vi "XYZ Stage Driver.vi"(11 "UI elements cluster":T1) -> (0 "error out (no error)":errorcluster)   [LabVIEW 2020]
uses:
  Global Variables/General Globals.vi
  Typedefs/HW config states enum.ctl
  Typedefs/XYZ stage states.ctl
  Global Variables/gl_UI Ctrl Refs.vi
  Globals/gl_XYZStage globals.vi
  Typedefs/Plane Mode.ctl
  Typedefs/Laser control knob.ctl
  Typedefs/PMT control knob.ctl
  Typedefs/XY Stage_Move.ctl
  Typedefs/Frame Size.ctl
  Typedefs/UI ctrl refs cluster.ctl
  Acquisition/Typedefs/Ref DAQ Param.ctl
  Typedefs/test_fpga_control.ctl
  User Interface/Misc/Biology Information.ctl
  User Interface/Misc/Experiment Type.ctl
panel:
  out "Interrupt loop itr":i32
  out "XYZ stage initialised":bool
  out "Motor driver loop itr":i32
  out "Command":T2
  out "Coordinates":cluster{"X":sgl, "Y":sgl, "Z":sgl}
  out "internal error cluster":errorcluster
  # "XYZ STAGE DRIVER"
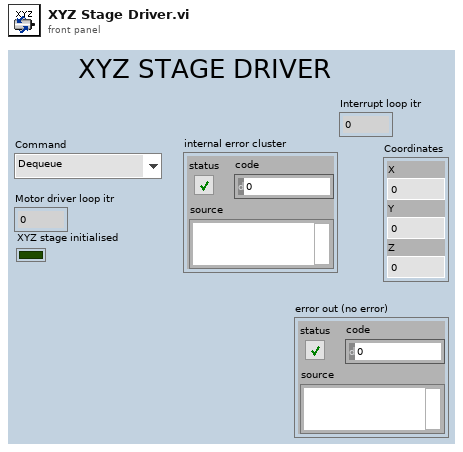
[diagram p1: front panel]
types:
  T1 = typedef "UI ctrl refs cluster.ctl" = cluster{"Top level VI path":path, "Top level VI ref":refnum<vi>, "User menu ref":refnum<k9>, "Sub Panel control":refnum<vi>, "Imaging Param Tab":refnum<vi>, "Occurrence-Start drivers":refnum<k4>, "Occurrence-Speed logging initialised":refnum<k4>, "Occurrence-XYZ stage initialised":refnum<k4>, "Exit button":refnum<vi>, "Status ind":refnum<vi>, "Set as origin":refnum<vi>, "Speed Logging":refnum<vi>, "Time Lapse":refnum<vi>, "Live Imaging":refnum<vi>, "AOL Z Stack":refnum<vi>, "Motor Z Stack":refnum<vi>, "Funct Acq button":refnum<vi>, "Hard Shutter":refnum<vi>, "Virtual Shutter":refnum<vi>, "Laser Power":refnum<vi>, "AOL Mode":refnum<vi>, "Frame Size":refnum<vi>, "Field of View":refnum<vi>, "Dwell Time":refnum<vi>, "Zoom":refnum<vi>, "AOL Z":refnum<vi>, "Objective":refnum<vi>, "Axis":refnum<vi>, "Paths & Names":refnum<vi>, "Experiment folder path (ind.)":refnum<vi>, "Last State (Ind.)":refnum<vi>, "Averages":refnum<vi>, "Angle (degrees)":refnum<vi>, "X centre":refnum<vi>, "Y centre":refnum<vi>, "Plane Mode":refnum<vi>, "# Planes":refnum<vi>, "Z Start":refnum<vi>, "Z Stop":refnum<vi>, "Z Step":refnum<vi>, "PMT 1":refnum<vi>, "PMT 2":refnum<vi>, "Stage XYZ Position":refnum<vi>, "Pockels@Z Start":refnum<vi>, "Pockels@Z Stop":refnum<vi>, "Obtain Z Start":refnum<vi>, "Obtain Z Stop":refnum<vi>, "Live stim.trig.period":refnum<vi>, "Live stim.trig.enable":refnum<vi>, "Movement Correction":refnum<vi>, "Load Reference Image":refnum<vi>, "XY Stage Move":refnum<vi>, "MovCor Cluster":refnum<vi>, "RefDAQParam":refnum<vi>, "Funct. Acq. Pockels Modulation":refnum<vi>, "Ref Laser Power":refnum<vi>, "Enable Video Recording":refnum<vi>, "Video Record-Live Imaging":refnum<vi>, "Video Record-Funct acq":refnum<vi>, "Reference Source":refnum<vi>, "AOL Z-stack Chirps Ready (ind)":refnum<vi>, "Target time between mov.cor. ref triggers (ms)":refnum<vi>, "Funct. Acq. Ref frame save":refnum<vi>, "Tracking button":refnum<vi>, "Show ref plots window":refnum<vi>, "Center freq ind (nm)":refnum<vi>, "Pickup mode (ind)":refnum<vi>, "Logging queue (ind)":refnum<vi>, "Back aperture power (ind.)":refnum<vi>, "Power after objective (ind.)":refnum<vi>, "Switch user":refnum<vi>, "Ls1 Conn. Status":refnum<vi>, "Ls1Tuning Status":refnum<vi>, "Ls1 Faults":refnum<vi>, "Ls1 Connection":refnum<vi>, "Ls1 Mode":refnum<vi>, "Ls1 POWER [mW]":refnum<vi>, "Ls1Shutter":refnum<vi>, "Ls1 Wavelength":refnum<vi>, "Ls1 Note":refnum<vi>, "Ls1 Confirm Wav":refnum<vi>, "Ls1 PreChrp Prism1":refnum<vi>, "Ls1 PreChrp Prism2":refnum<vi>, "Ls1 wav top Ind":refnum<vi>, "Ls1 power top Ind":refnum<vi>, "Ls1 Pump peak Hold":refnum<vi>, "Ls1 Status Ind":refnum<vi>, "Ls1 wav cancel":refnum<vi>, "Experiment Type":refnum<vi>, "Biology Information":refnum<vi>, "Camera recording status":refnum<vi>, "Optimise Obj. Pos.":refnum<vi>}
  T2 = typedef "XYZ stage states.ctl" = enum16{"Dequeue", "Initialize", "Read Position", "Read Speed Setting", "Move", "Set Max Speed", "Reset Axis", "Stop all movement"}
  T3 = typedef "HW config states enum.ctl" = enum16{"Load from file", "Save to file", "Save backup", "Write all", "Read all", "Write XY stage settings", "Write DAQ FPGA settings", "Write Control FPGA settings", "Write Phys Channels", "Write System Config", "Write HW Config", "Save System Config", "Save HW Config", "Clear", "Compare from file"}
  T4 = typedef "Hardware Configuration settings.ctl" = cluster{"Dev. PC":bool, "Swap XY on stage":bool, "No of AOD":u8, "MC Supported":bool, "Axial MC":bool, "Computer MAC address":string, "Externalise Triggers":bool, "Trigger HW config":T5, "DAQmx Chan":T6, "XYZ Stage Control Config":T7, "XY stage available":bool, "XY Comms Config Cluster":T8, "Y stage available":bool, "Y Comms Config Cluster":T8, "Z stage available":bool, "Z Comms Config Cluster ":T8, "Encoder available":bool, "Encoder":T10, "VidRec available":bool, "Cam VidRec":T11, "Laser Power Control HW config":T12, "Laser 1 available":bool, "Laser 1 config cluster":T13, "Prechirper 1 available":bool, "Prechirper 1 config cluster":T14, "Control system.FPGA available?":bool, "Control Sys. HW config":T15, "DAQ FPGA HW Config":T16, "PMT Control Voltage Limits":T20}
  T5 = typedef "Triggers HW config.ctl" = cluster{"Available Device List":i32, "Device Address":string}
  T6 = typedef "DAQmx physical channels cluster.ctl" = cluster{"Pockels AO":tag, "Hard shutter AO":tag, "PMT AOs":tag, "Galvo AOs":tag, "Power meter AI":tag}
  T7 = typedef "XYZControlConfig.ctl" = enum16{"None", "XYZ", "XY-Z", "X-Y-Z", "Z"}
  T8 = typedef "Peripherals comms config cluster.ctl" = cluster{"Name":string, "Device Address":string, "Port ":u16, "Baudrate":i32, "Comms Type":T9}
  T9 = typedef "Comms Type.ctl" = enum16{"GPIB-IEEE488", "Serial-RS232", "Serial-RS485", "Serial-RS422", "Serial-USB", "Ethernet-TCP/IP", "Ethernet-UDP"}
  T10 = typedef "Encoder config cluster.ctl" = cluster{"IP address":string, "Port":u16, "Wheel radius (cm)":dbl, "Encoder Trigger":tag}
  T11 = typedef "Cam VidRec HW config setup cluster.ctl" = cluster{"DO flag-Video record":tag, "DO flag-Trial start":tag}
  T12 = typedef "Laser Power Control HW config.ctl" = cluster{"Laser Power Control":string, "Laser Power Modulation Control":enum16{"NI", "FPGA"}}
  T13 = typedef "Laser 1 config cluster.ctl" = cluster{"COM port":refnum<visa-resource-name>, "Baud Rate":i32, "Type":string}
  T14 = typedef "PreChirper 1 config cluster.ctl" = cluster{"Type":string, "Baud Rate":i32, "COM port":refnum<visa-resource-name>}
  T15 = typedef "Control Sys HW config cluster.ctl" = cluster{"Control system.FPGA Type":enum16{"Virtex 5", "Virtex 7"}, "Control system.Network adapter name":string, "Control system.MAC address":string, "Control system.Ethernet Port":u32, "Control system.Ethernet Port Opened":bool}
  T16 = typedef "DAQ FPGA HW config cluster.ctl" = cluster{"FGPA Ref":T17, "Target":T18, "input card type":T19}
  T17 = typedef "FPGA Ref.ctl" = refnum<k20>
  T18 = typedef "nirio_resource_hc.ctl" = tag
  T19 = typedef "FPGA input type AC-DC.ctl" = enum16{"AC Card", "DC Card"}
  T20 = typedef "PMT Control Voltage limits.ctl" = cluster{"Lower Limit":dbl, "Upper Limit":dbl}
  T21 = typedef "XYZ stage data.ctl" = cluster{"Command":T2, "Channel":T22, "X":sgl, "Y":sgl, "Z":sgl, "Speed":i32, "Zero":bool, "Use acknowledgement?":bool}
  T22 = typedef "XYZ channel ring.ctl" = string
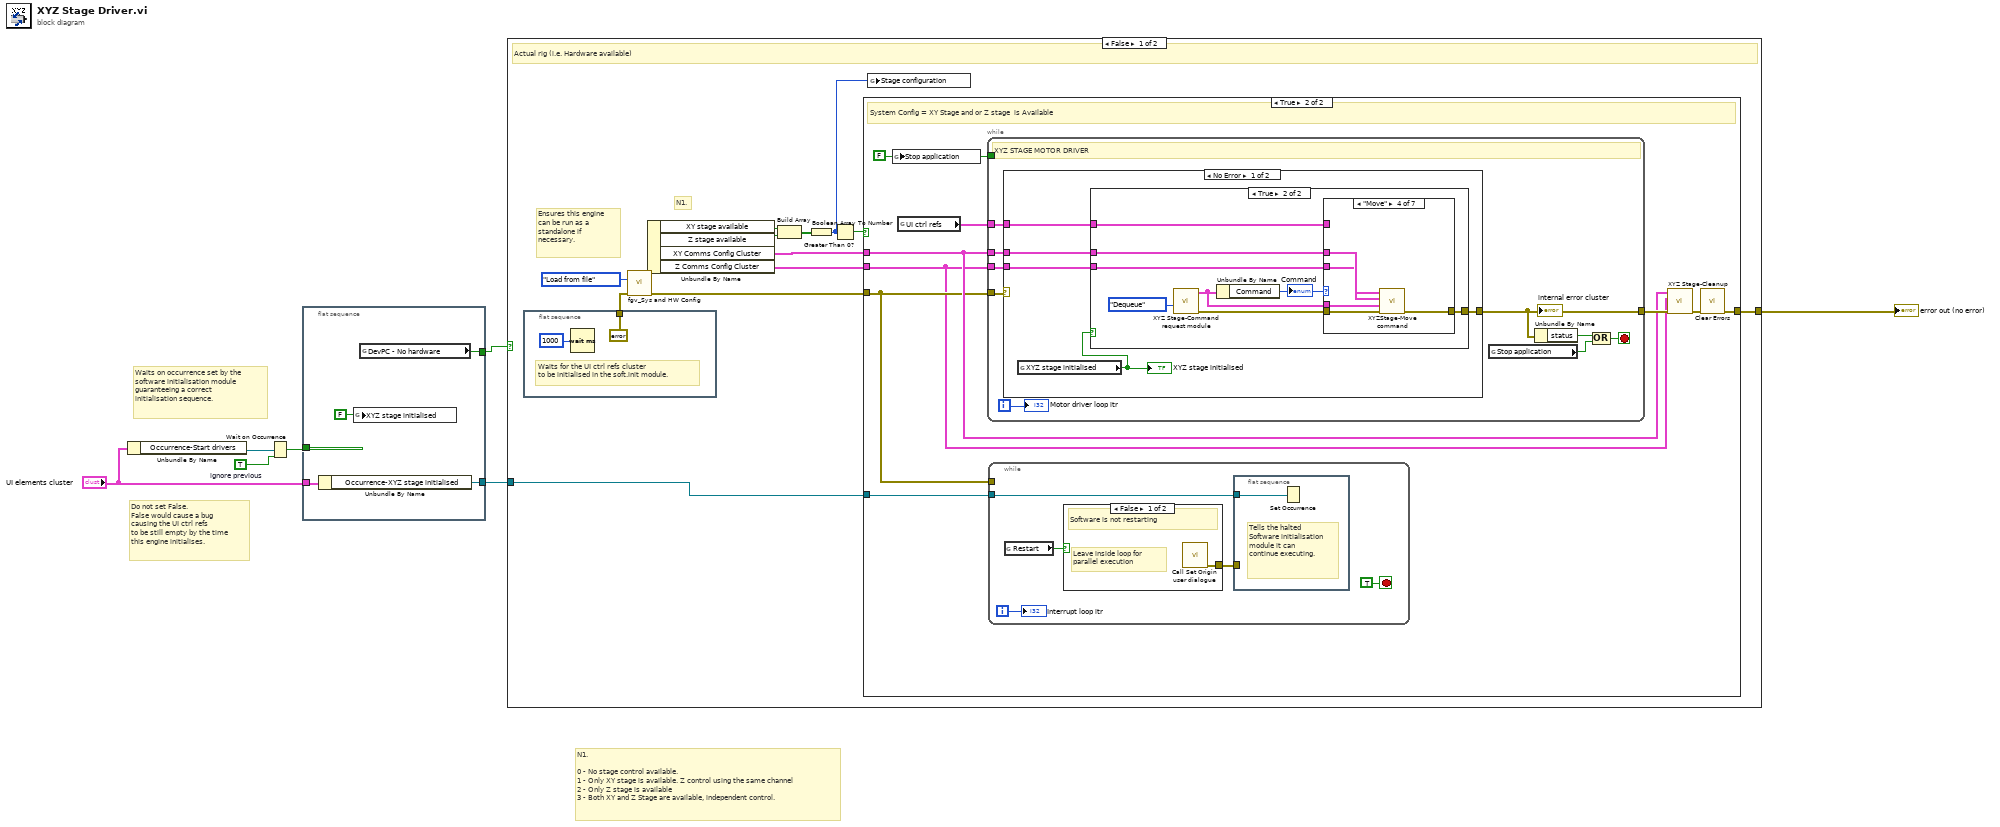
[diagram p0: block diagram]
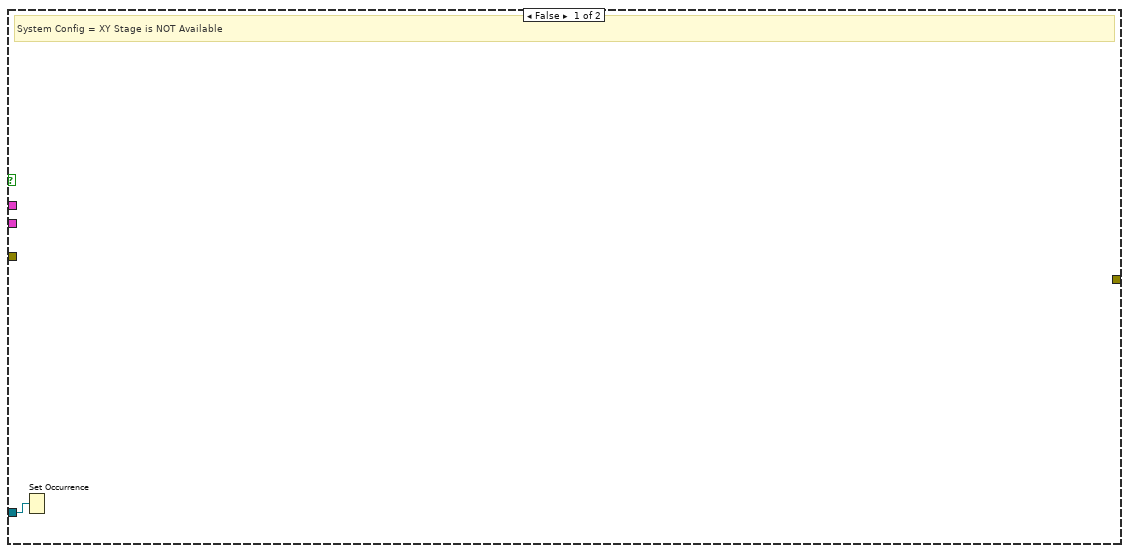
[diagram p2: hidden frame]
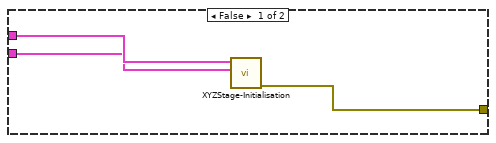
[diagram p4: hidden frame]
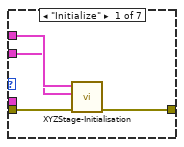
[diagram p5: hidden frame]
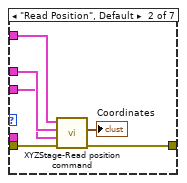
[diagram p6: hidden frame]
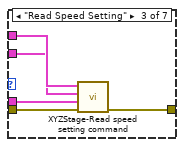
[diagram p7: hidden frame]
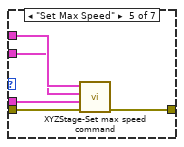
[diagram p8: hidden frame]
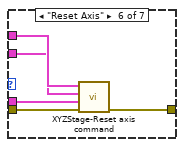
[diagram p9: hidden frame]
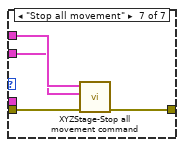
[diagram p10: hidden frame]
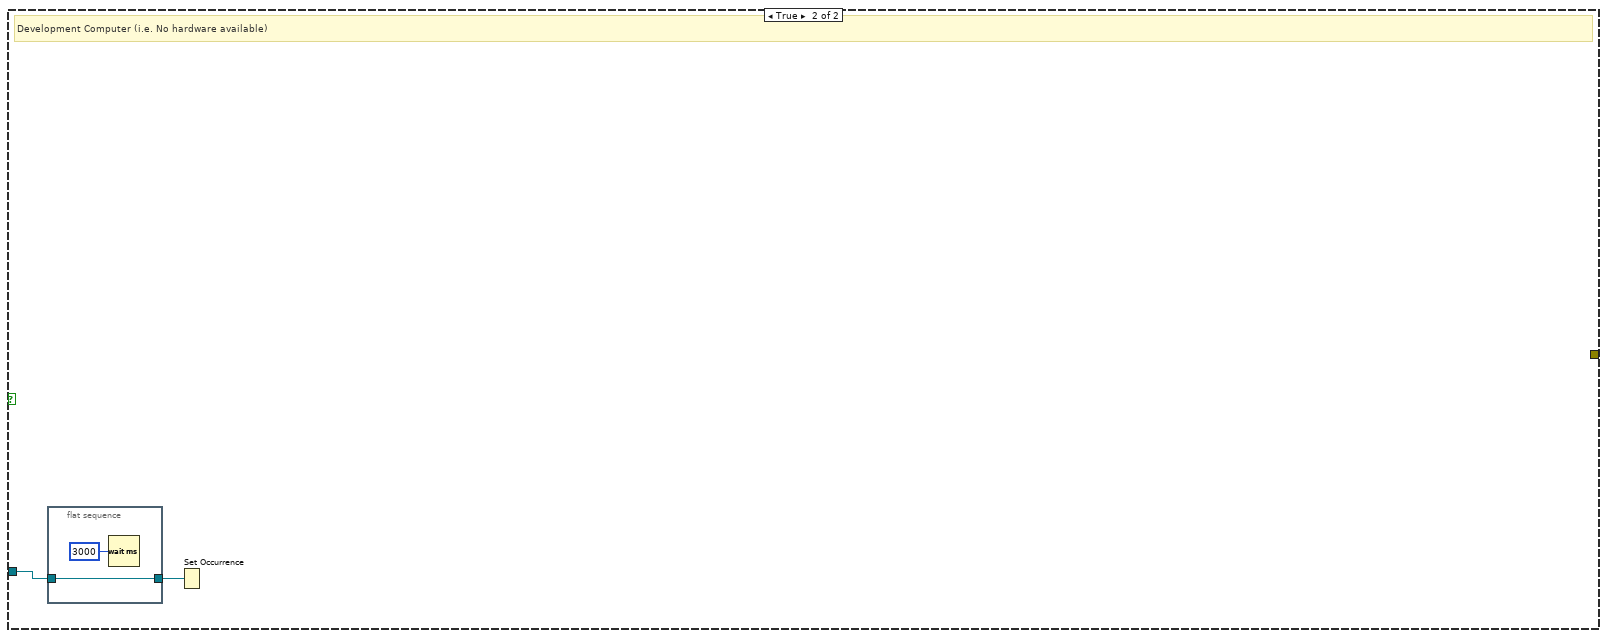
[diagram p12: hidden frame]
diagram:
  w3 = TRUE  # ignore previous
  # "N1. \n\n0 - No stage control available.\n1 - Only XY stage is available. Z control using the same channel\n2 - Only Z stage is available\n3 - Both XY and Z Stage are available, independent control."
  # "Do not set False.\nFalse would cause a bug\ncausing the UI ctrl refs\nto be still empty by the time\nthis engine initialises."
  # "Waits on occurrence set by the software initialisation module guaranteeing a correct initialisation sequence."
  n1 = Unbundle By Name("UI elements cluster") -> ("Occurrence-Start drivers"=w2:refnum<k4>)
  n2 = Wait on Occurrence(1:w3, 2:w2) -> (0:w4:bool)  [unwired: 1 in]
  n3 = flat-sequence {
    tunnel: [w11] -> w1
    tunnel: "UI elements cluster" -> [w10]
    tunnel: [w9] -> w6
    tunnel: w4 -> [_]
    frame #0 {
      n4 = Unbundle By Name(w10) -> ("Occurrence-XYZ stage initialised"=w9:refnum<k4>)
      n5 = global write "gl_XYZStage globals.vi" "XYZ stage initialised"(FALSE ("XYZ stage initialised")) -> ()
      n6 = global read "General Globals.vi" "DevPC - No hardware"() -> (w11:bool)
    }
  }
  n7 = case shown="False" w1 {
    tunnel: [w20 _] -> w7
    tunnel: w6 -> [w18 w105]
    frame False {
      # "N1."
      # "Ensures this engine can be run as a standalone if necessary."
      # "Actual rig (i.e. Hardware available)"
      n8 = flat-sequence {
        tunnel: [errorcluster {"status"=FALSE, "code"=0, "source"=""} ("error in (no error)")] -> w19
        frame #0 {
          # "Waits for the UI ctrl refs cluster\nto be initialised in the soft.init module."
          n9 = Wait (ms)(milliseconds to wait=u32 1000) -> ()  [unwired: 1 out]
        }
      }
      n10 = call "fgv_Sys and HW Config.vi"("Function"=HW_config_states_enum."Load from file", "error in (no error)"=w19) -> ("error out"=w21:errorcluster, "Hardware Configuration OUT"=w22:T4)  [unwired: 7 in, 1 out]
      n11 = Unbundle By Name(w22) -> ("XY stage available"=w16:bool, "Z stage available"=w15:bool, "XY Comms Config Cluster"=w24:T8, "Z Comms Config Cluster"=w17:T8)
      n12 = Build Array(w16, w15) -> (w14:bool[])
      n13 = Boolean Array To Number(Boolean array=w14) -> (number=w12:u32)
      n14 = Greater Than 0?(x=w12) -> (x > 0?=w13:bool)
      n15 = case shown="True" w13 {
        tunnel: w24 -> [_ w35]
        tunnel: w18 -> [w27 w34]
        tunnel: w21 -> [_ w32]
        tunnel: [_ w30] -> w20
        tunnel: w17 -> [_ w28]
        frame False {
          # "System Config = XY Stage is NOT Available"
          n16 = Set Occurrence(w27) -> ()
        }
        frame True {
          w33 = FALSE ("Stop application")
          # "System Config = XY Stage and or Z stage  is Available"
          n17 = global write "General Globals.vi" "Stop application"(w33) -> ()
          n18 = global read "gl_UI Ctrl Refs.vi" "UI ctrl refs"() -> (w29:T1)
          n19 = while {
            tunnel: w32 -> [w49]
            tunnel: [w47] -> w36
            tunnel: w35 -> [w50]
            tunnel: w33 -> [_]
            tunnel: w29 -> [w46]
            tunnel: w28 -> [w44]
            i -> [w45]
            stop <- w52 stop-if-true
            # "XYZ STAGE MOTOR DRIVER"
            n20 = case shown="No Error" w49 {
              selector: w49 -> [_ w103]
              tunnel: [w56 w103] -> w47
              tunnel: w50 -> [w57 _]
              tunnel: w46 -> [w54 _]
              tunnel: w44 -> [w53 _]
              frame No Error {
                n21 = global read "gl_XYZStage globals.vi" "XYZ stage initialised"() -> (w55:bool)
                "XYZ stage initialised" <- w55
                n22 = case shown="True" w55 {
                  tunnel: w57 -> [w60 w68]
                  tunnel: [w59 w67] -> w56
                  tunnel: w54 -> [_ w62]
                  tunnel: w53 -> [w58 w61]
                  frame False {
                    n23 = call "XYZStage-Initialisation.vi"("Z Stage"=w58, "XY Stage"=w60) -> ("Error Out"=w59:errorcluster)  [unwired: 8 in, 1 out]
                  }
                  frame True {
                    n24 = call "XYZ Stage-Command request module.vi"("Command"=XYZ_stage_states."Dequeue") -> ("error out"=w65:errorcluster, "XYZ Stage dequeued data"=w64:T21)  [unwired: 6 in, 3 out]
                    n25 = Unbundle By Name(w64) -> ("Command"=w66:T2)
                    "Command" <- w66
                    n26 = case shown="\"Move\"" w66 {
                      tunnel: w68 -> [w71 w77 w80 w86 w91 w95 w100]
                      tunnel: w64 -> [_ _ w81 w85 w90 w96 _]
                      tunnel: w65 -> [w72 w78 w83 w88 w93 w97 w101]
                      tunnel: [w70 w76 w82 w87 w92 w98 w102] -> w67
                      tunnel: w62 -> [_ w74 _ _ _ _ _]
                      tunnel: w61 -> [w69 w73 w79 w84 w89 w94 w99]
                      frame "Initialize" {
                        n27 = call "XYZStage-Initialisation.vi"("Error In"=w72, "Z Stage"=w69, "XY Stage"=w71) -> ("Error Out"=w70:errorcluster)  [unwired: 7 in, 1 out]
                      }
                      frame "Read Position", Default {
                        n28 = call "XYZStage-Read position command.vi"("error in (no error)"=w78, "Z Stage"=w73, "XY Stage config cluster"=w77, "UI ctrl refs"=w74) -> ("error out"=w76:errorcluster, "Coordinates"=→"Coordinates":cluster{"X":sgl, "Y":sgl, "Z":sgl})  [unwired: 6 in]
                      }
                      frame "Read Speed Setting" {
                        n29 = call "XYZStage-Read speed setting command.vi"("error in (no error)"=w83, "XYZ Stage data to queue"=w81, "Z Stage"=w79, "XY Stage config cluster"=w80) -> ("error out"=w82:errorcluster)  [unwired: 7 in]
                      }
                      frame "Move" {
                        n30 = call "XYZStage-Move command.vi"("Error In"=w88, "XYZ Stage data"=w85, "Z Stage"=w84, "XYZ Stage config"=w86) -> ("Error Out"=w87:errorcluster)  [unwired: 6 in, 1 out]
                      }
                      frame "Set Max Speed" {
                        n31 = call "XYZStage-Set max speed command.vi"("Error In"=w93, "XYZ Stage data"=w90, "Z Stage"=w89, "XYZ Stage config"=w91) -> ("Error Out"=w92:errorcluster)  [unwired: 7 in]
                      }
                      frame "Reset Axis" {
                        n32 = call "XYZStage-Reset axis command.vi"("error in (no error)"=w97, "XYZ Stage dequeued data"=w96, "Z Stage"=w94, "XY Stage"=w95) -> ("error out"=w98:errorcluster)  [unwired: 7 in]
                      }
                      frame "Stop all movement" {
                        n33 = call "XYZStage-Stop all movement command.vi"("Error In"=w101, "Z Stage"=w99, "XYZ Stage config"=w100) -> ("Error Out"=w102:errorcluster)  [unwired: 7 in, 1 out]
                      }
                    }
                  }
                }
              }
              frame Error {
              }
            }
            "internal error cluster" <- w47
            n34 = global read "General Globals.vi" "Stop application"() -> (w48:bool)
            n35 = Unbundle By Name(w47) -> ("status"=w51:bool)
            n36 = Compound Arithmetic op=OR(w51, w48) -> (w52:bool)
            "Motor driver loop itr" <- w45
          }
          n37 = while {
            tunnel: w32 -> [_]
            tunnel: w34 -> [w39]
            i -> [w37]
            stop <- TRUE stop-if-true
            n38 = global read "General Globals.vi" "Restart"() -> (w38:bool)
            n39 = case shown="False" w38 {
              tunnel: [w42 _] -> w40
              frame False {
                # "Leave inside loop for parallel execution"
                # "Software is not restarting"
                n40 = call "Call Set Origin user dialogue.vi"() -> ("error out"=w42:errorcluster)  [unwired: 11 in]
              }
              frame True {
                # "Software Restarting"
              }
            }
            n41 = flat-sequence {
              tunnel: w40 -> [_]
              tunnel: w39 -> [w43]
              frame #0 {
                # "Tells the halted Software initialisation\nmodule it can continue executing."
                n42 = Set Occurrence(w43) -> ()
              }
            }
            "Interrupt loop itr" <- w37
          }
          n43 = call "XYZ Stage-Cleanup.vi"("error in (no error)"=w36, "Z Stage config cluster"=w28, "XY Stage config cluster"=w35) -> ("error out"=w31:errorcluster)  [unwired: 8 in]
          n44 = call <vilib>:"Clear Errors.vi"("error in (no error)"=w31) -> ("error out"=w30:errorcluster)  [unwired: 5 in, 1 out]
        }
      }
      n45 = global write "General Globals.vi" "Stage configuration"(w12) -> ()
    }
    frame True {
      # "Development Computer (i.e. No hardware available)"
      n46 = flat-sequence {
        tunnel: w105 -> [w107]
        tunnel: [w107] -> w104
        frame #0 {
          n47 = Wait (ms)(milliseconds to wait=u32 3000) -> ()  [unwired: 1 out]
        }
      }
      n48 = Set Occurrence(w104) -> ()
    }
  }
  "error out (no error)" <- w7
